vi "SetProxy.vi"(8 "error in (no error)":errorcluster, 10 "Proxy":refnum<class "Subject.lvclass">, 11 "Subject in":refnum<class "Subject.lvclass">) -> (0 "error out":errorcluster, 3 "Subject out":refnum<class "Subject.lvclass">)   [LabVIEW 2014, in "forcible Proxy.lvlib" / "Subject.lvclass"]
uses:
  Subject.lvclass
  Subject.lvclass/Subject.ctl
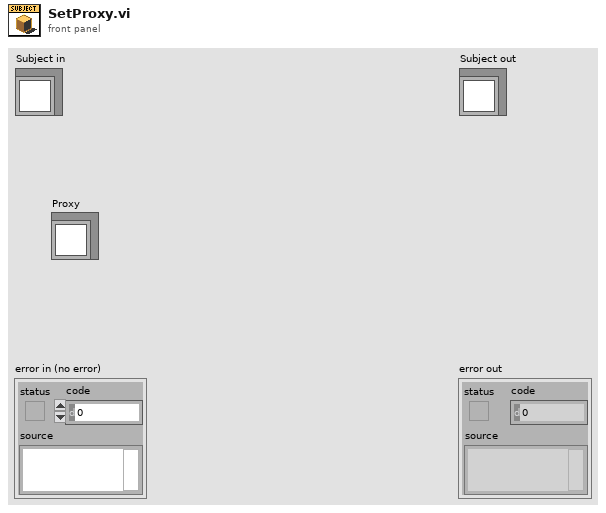
[diagram p1: front panel]
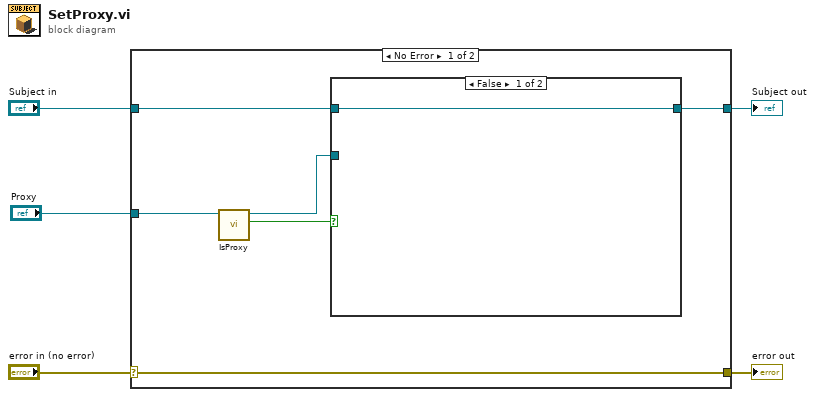
[diagram p0: block diagram]
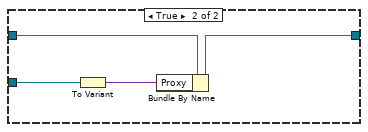
[diagram p2: hidden frame]
diagram:
  n1 = case shown="No Error" "error in (no error)" {
    selector: "error in (no error)" -> [w11 w18]
    tunnel: [w11 w18] -> w4
    tunnel: [w9 w17] -> w2
    tunnel: "Subject in" -> [w8 w17]
    tunnel: "Proxy" -> [w10 _]
    frame No Error {
      n2 = call-dynamic "IsProxy.vi"("Subject in"=w10) -> ("isProxy?"=w7:bool, "Subject out"=w6:refnum<class "Subject.lvclass">)  [unwired: 8 in, 1 out]
      n3 = case shown="False" w7 {
        tunnel: [w12 w15] -> w9
        tunnel: w8 -> [w12 w16]
        tunnel: w6 -> [_ w14]
        frame False {
        }
        frame True {
          n4 = To Variant(anything=w14) -> (Variant=w13:variant)
          n5 = Bundle By Name(cluster=w16, "Proxy"=w13) -> (w15:refnum<class "Subject.lvclass">)
        }
      }
    }
    frame Error {
    }
  }
  "error out" <- w4
  "Subject out" <- w2
